vi "Measurement.SetConfiguration.vi"(8 "error in (no error)":errorcluster, 10 "Configuration":variant, 11 "Measurement.Free in":refnum<class "Measurement.Free.lvclass">) -> (0 "error out":errorcluster, 3 "Measurement.Free out":refnum<class "Measurement.Free.lvclass">)   [LabVIEW 2017, in "Measurement.Free.lvclass"]
uses:
  Measurement.Free.lvclass
  Typedefs/Configuration--Cluster.ctl
  Typedefs/Configuration.Hardware--Cluster.ctl
  Measurement/Typedefs/Configuration.SMU--Cluster.ctl
  SMU/Typedefs/Configuration--Cluster.ctl
  Measurement/Typedefs/Configuration.LIA--Cluster.ctl
  LIA/Typedefs/Configuration--Cluster.ctl
  Measurement/Typedefs/Configuration.OPM--Cluster.ctl
  OPM/Typedefs/Configuration--Cluster.ctl
  Measurement/Typedefs/Configuration.OPA--Cluster.ctl
  OPA/Typedefs/Configuration--Cluster.ctl
  SMU/SMU.lvclass
  Measurement/Measurement.lvclass
  LIA/LIA.lvclass
  OPM/OPM.lvclass
  OPA/OPA.lvclass
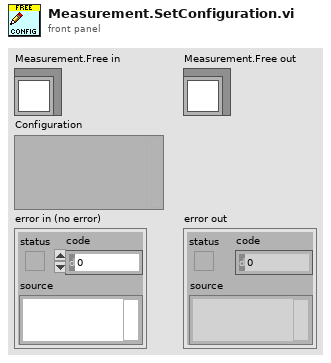
[diagram p1: front panel]
types:
  T1 = typedef "Measurement.Free.lvclass/Configuration--Cluster.ctl" = cluster{"Measurement.Type":enum16{"Free", "I/V Curve", "Wavelength sweeping", "Photocurrent mapping"}, "Hardware":T2}
  T2 = typedef "Measurement.Free.lvclass/Configuration.Hardware--Cluster.ctl" = cluster{"SMU":T3, "LIA":T5, "OPM":T7, "OPA":T9}
  T3 = typedef "Measurement.lvclass/Configuration.SMU--Cluster.ctl" = cluster{"Enable":bool, "SMU Model":string, "Configuration":T4}
  T4 = typedef "SMU.lvclass/Configuration--Cluster.ctl" = cluster{"VISA Resource":string, "Channel":string}
  T5 = typedef "Measurement.lvclass/Configuration.LIA--Cluster.ctl" = cluster{"Enable":bool, "LIA Model":string, "Configuration":T6}
  T6 = typedef "LIA.lvclass/Configuration--Cluster.ctl" = cluster{"VISA Resource":string}
  T7 = typedef "Measurement.lvclass/Configuration.OPM--Cluster.ctl" = cluster{"Enable":bool, "OPM Model":string, "Configuration":T8}
  T8 = typedef "OPM.lvclass/Configuration--Cluster.ctl" = cluster{"VISA Resource":string}
  T9 = typedef "Measurement.lvclass/Configuration.OPA--Cluster.ctl" = cluster{"Enable":bool, "OPA Model":string, "Configuration":T10}
  T10 = typedef "OPA.lvclass/Configuration--Cluster.ctl" = cluster{"Serial Number":string}
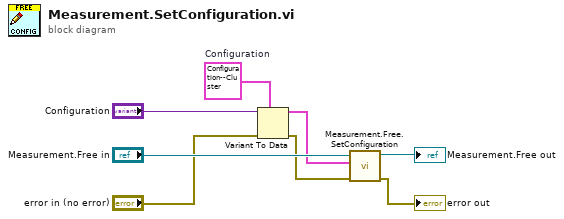
[diagram p0: block diagram]
diagram:
  w7 = T1 {"Measurement.Type"=enum."Free", "Hardware"={"SMU"={"Enable"=FALSE, "SMU Model"="", "Configuration"={"VISA Resource"="", "Channel"=""}}, "LIA"={"Enable"=FALSE, "LIA Model"="", "Configuration"={"VISA Resource"=""}}, "OPM"={"Enable"=FALSE, "OPM Model"="", "Configuration"={"VISA Resource"=""}}, "OPA"={"Enable"=FALSE, "OPA Model"="", "Configuration"={"Serial Number"=""}}}}  # Configuration
  n1 = Variant To Data(error in="error in (no error)", type=w7, Variant="Configuration") -> (data=w3:T1, error out=w4:errorcluster)
  n2 = call "Measurement.Free.SetConfiguration.vi"("error in (no error)"=w4, "Configuration"=w3, "Measurement.Free"="Measurement.Free in") -> ("error out"=→"error out":errorcluster, "Measurement.Free out"=→"Measurement.Free out":refnum<class "Measurement.Free.lvclass">)  [unwired: 7 in]
